vi "Single to Double Backslash.vi"(1 "input":string caption="Eingang") -> (0 "output":string caption="Ausgang")   [LabVIEW 2009]
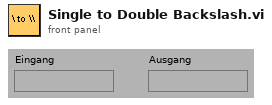
[diagram p1: front panel]
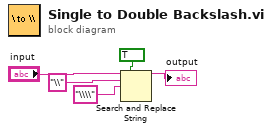
[diagram p0: block diagram]
diagram:
  n1 = Search and Replace String(replace all?=TRUE ("replace all? (F)"), input string="input", search string="\\" ("regular expression"), replace string="\\\\") -> (result string=→"output":string)  [unwired: 4 in, 3 out]
